vi "Change temperature with fixed current.vi"() -> ()   [LabVIEW 2013]
uses:
  <vilib>/Analysis/NI_AALBase.lvlib
panel:
  out "Variance":dbl[](array[numeric]) format="%#.2g"
  out "SD":dbl[](array[numeric]) format="%#.2g"
  out "Mean":dbl[](array[numeric]) format="%#.2f"
  out "variance":dbl format="%0.2f"
  out "standard deviation":dbl format="%0.2f"
  out "mean":dbl format="%0.2f"
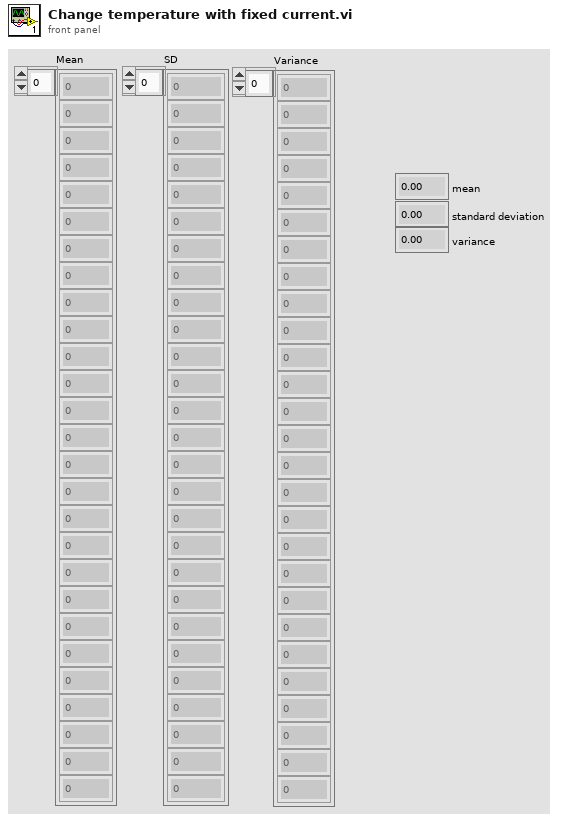
[diagram p1: front panel]
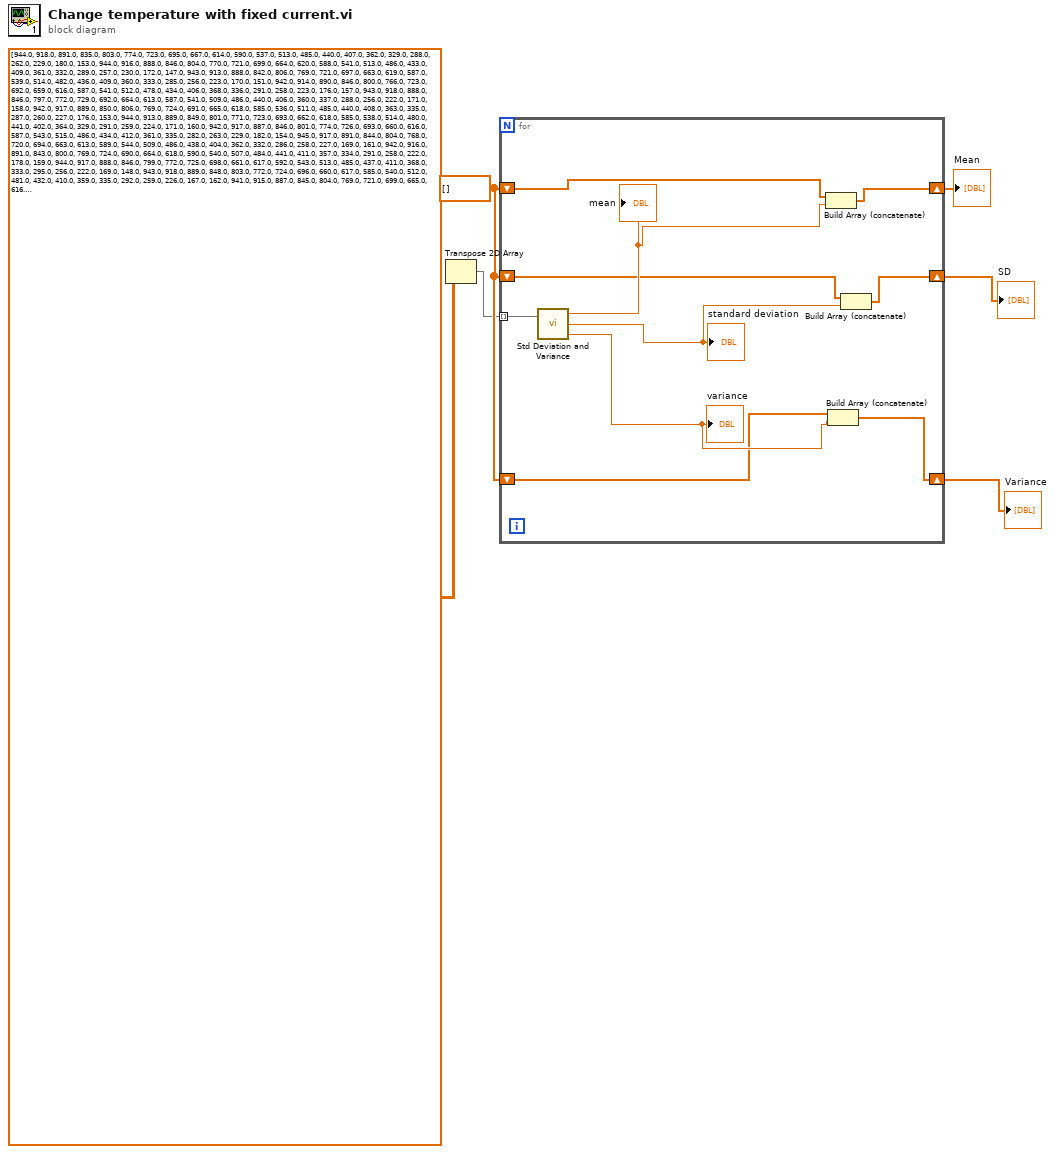
[diagram p0: block diagram]
diagram:
  w6 = dbl[] []
  n1 = Transpose 2D Array(2D array=dbl[][] [[944.0, 918.0, 891.0, 835.0, 803.0, 774.0, 723.0, 695.0, 667.0, 614.0, 590.0, 537.0, 513.0, 485.0, 440.0, 407.0, 362.0, 329.0, 288.0, 262.0, 229.0, 180.0, 153.0], [944.0, 916.0, 888.0, 846.0, 804.0, 770.0, 721.0, 699.0, 664.0, 620.0, 588.0, 541.0, 513.0, 486.0, 433.0, 409.0, 361.0, 332.0, 289.0, 257.0, 230.0, 172.0, 147.0], [943.0, 913.0, 888.0, 842.0, 806.0, 769.0, 721.0, 697.0, 663.0, 619.0, 587.0, 539.0, 514.0, 482.0, 436.0, 409.0, 360.0, 333.0, 285.0, 256.0, 223.0, 170.0, 151.0], [942.0, 914.0, 890.0, 846.0, 800.0, 766.0, 723.0, 692.0, 659.0, 616.0, 587.0, 541.0, 512.0, 478.0, 434.0, 406.0, 368.0, 336.0, 291.0, 258.0, 223.0, 176.0, 157.0], [943.0, 918.0, 888.0, 846.0, 797.0, 772.0, 729.0, 692.0, 664.0, 613.0, 587.0, 541.0, 509.0, 486.0, 440.0, 406.0, 360.0, 337.0, 288.0, 256.0, 222.0, 171.0, 158.0], [942.0, 917.0, 889.0, 850.0, 806.0, 769.0, 724.0, 691.0, 665.0, 618.0, 585.0, 536.0, 511.0, 485.0, 440.0, 408.0, 363.0, 335.0, 287.0, 260.0, 227.0, 176.0, 153.0], [944.0, 913.0, 889.0, 849.0, 801.0, 771.0, 723.0, 693.0, 662.0, 618.0, 585.0, 538.0, 514.0, 480.0, 441.0, 402.0, 364.0, 329.0, 291.0, 259.0, 224.0, 171.0, 160.0], [942.0, 917.0, 887.0, 846.0, 801.0, 774.0, 726.0, 693.0, 660.0, 616.0, 587.0, 543.0, 515.0, 486.0, 434.0, 412.0, 361.0, 335.0, 282.0, 263.0, 229.0, 182.0, 154.0], [945.0, 917.0, 891.0, 844.0, 804.0, 768.0, 720.0, 694.0, 663.0, 613.0, 589.0, 544.0, 509.0, 486.0, 438.0, 404.0, 362.0, 332.0, 286.0, 258.0, 227.0, 169.0, 161.0], [942.0, 916.0, 891.0, 843.0, 800.0, 769.0, 724.0, 690.0, 664.0, 618.0, 590.0, 540.0, 507.0, 484.0, 441.0, 411.0, 357.0, 334.0, 291.0, 258.0, 222.0, 178.0, 159.0], [944.0, 917.0, 888.0, 846.0, 799.0, 772.0, 725.0, 698.0, 661.0, 617.0, 592.0, 543.0, 513.0, 485.0, 437.0, 411.0, 368.0, 333.0, 295.0, 256.0, 222.0, 169.0, 148.0], [943.0, 918.0, 889.0, 848.0, 803.0, 772.0, 724.0, 696.0, 660.0, 617.0, 585.0, 540.0, 512.0, 481.0, 432.0, 410.0, 359.0, 335.0, 292.0, 259.0, 226.0, 167.0, 162.0], [941.0, 915.0, 887.0, 845.0, 804.0, 769.0, 721.0, 699.0, 665.0, 616.0, 588.0, 540.0, 512.0, 482.0, 437.0, 406.0, 367.0, 332.0, 286.0, 262.0, 217.0, 178.0, 159.0], [941.0, 916.0, 891.0, 848.0, 805.0, 771.0, 724.0, 693.0, 664.0, 613.0, 586.0, 535.0, 514.0, 483.0, 441.0, 407.0, 365.0, 335.0, 285.0, 262.0, 223.0, 180.0, 155.0], [942.0, 916.0, 887.0, 849.0, 800.0, 773.0, 722.0, 691.0, 667.0, 616.0, 589.0, 544.0, 509.0, 478.0, 442.0, 411.0, 359.0, 337.0, 287.0, 257.0, 227.0, 177.0, 157.0], [942.0, 918.0, 888.0, 845.0, 800.0, 769.0, 724.0, 695.0, 665.0, 622.0, 587.0, 541.0, 507.0, 481.0, 437.0, 408.0, 368.0, 336.0, 289.0, 258.0, 225.0, 174.0, 155.0], [941.0, 915.0, 887.0, 845.0, 806.0, 769.0, 726.0, 697.0, 663.0, 617.0, 588.0, 543.0, 512.0, 482.0, 443.0, 406.0, 360.0, 336.0, 285.0, 260.0, 228.0, 163.0, 155.0], [942.0, 918.0, 890.0, 845.0, 804.0, 768.0, 722.0, 691.0, 664.0, 617.0, 582.0, 543.0, 513.0, 484.0, 440.0, 407.0, 359.0, 335.0, 292.0, 260.0, 224.0, 179.0, 151.0], [940.0, 915.0, 890.0, 849.0, 803.0, 771.0, 725.0, 690.0, 663.0, 617.0, 588.0, 542.0, 509.0, 482.0, 434.0, 410.0, 365.0, 337.0, 289.0, 257.0, 226.0, 176.0, 155.0], [942.0, 919.0, 890.0, 846.0, 805.0, 771.0, 728.0, 690.0, 664.0, 613.0, 590.0, 543.0, 510.0, 475.0, 433.0, 410.0, 361.0, 336.0, 287.0, 253.0, 228.0, 173.0, 152.0], [944.0, 916.0, 889.0, 850.0, 804.0, 771.0, 724.0, 694.0, 662.0, 619.0, 589.0, 543.0, 505.0, 485.0, 441.0, 407.0, 369.0, 342.0, 285.0, 261.0, 224.0, 168.0, 157.0], [942.0, 915.0, 888.0, 847.0, 804.0, 770.0, 725.0, 693.0, 667.0, 615.0, 589.0, 539.0, 513.0, 483.0, 434.0, 405.0, 367.0, 328.0, 294.0, 262.0, 228.0, 176.0, 149.0], [941.0, 914.0, 887.0, 841.0, 803.0, 769.0, 723.0, 691.0, 665.0, 617.0, 585.0, 541.0, 516.0, 483.0, 441.0, 407.0, 360.0, 338.0, 289.0, 259.0, 219.0, 175.0, 150.0], [943.0, 916.0, 890.0, 849.0, 804.0, 769.0, 721.0, 696.0, 665.0, 619.0, 589.0, 540.0, 513.0, 484.0, 441.0, 411.0, 368.0, 331.0, 288.0, 249.0, 218.0, 183.0, 150.0], [945.0, 919.0, 888.0, 845.0, 799.0, 773.0, 720.0, 695.0, 662.0, 618.0, 588.0, 540.0, 515.0, 484.0, 440.0, 405.0, 365.0, 331.0, 293.0, 256.0, 218.0, 163.0, 155.0], [943.0, 917.0, 890.0, 844.0, 804.0, 770.0, 724.0, 692.0, 664.0, 618.0, 588.0, 533.0, 512.0, 484.0, 437.0, 414.0, 356.0, 331.0, 290.0, 253.0, 223.0, 163.0, 152.0], [943.0, 916.0, 889.0, 846.0, 804.0, 774.0, 723.0, 694.0, 664.0, 613.0, 587.0, 537.0, 506.0, 484.0, 432.0, 412.0, 367.0, 340.0, 282.0, 255.0, 229.0, 175.0, 154.0], [941.0, 916.0, 891.0, 848.0, 801.0, 770.0, 726.0, 696.0, 661.0, 617.0, 587.0, 541.0, 512.0, 477.0, 439.0, 406.0, 365.0, 339.0, 285.0, 259.0, 221.0, 164.0, 152.0], [941.0, 914.0, 890.0, 848.0, 804.0, 769.0, 724.0, 694.0, 660.0, 616.0, 587.0, 546.0, 514.0, 483.0, 434.0, 412.0, 362.0, 331.0, 286.0, 252.0, 231.0, 182.0, 156.0], [944.0, 916.0, 890.0, 846.0, 804.0, 772.0, 724.0, 693.0, 661.0, 619.0, 586.0, 544.0, 515.0, 483.0, 440.0, 408.0, 365.0, 336.0, 290.0, 254.0, 226.0, 172.0, 156.0], [943.0, 917.0, 890.0, 848.0, 805.0, 770.0, 722.0, 695.0, 663.0, 617.0, 585.0, 543.0, 513.0, 480.0, 436.0, 406.0, 365.0, 336.0, 290.0, 257.0, 226.0, 178.0, 150.0], [942.0, 917.0, 888.0, 845.0, 801.0, 774.0, 723.0, 696.0, 665.0, 615.0, 589.0, 541.0, 512.0, 484.0, 444.0, 410.0, 363.0, 338.0, 289.0, 257.0, 221.0, 179.0, 150.0], [942.0, 915.0, 890.0, 845.0, 803.0, 769.0, 726.0, 695.0, 664.0, 613.0, 587.0, 534.0, 511.0, 485.0, 442.0, 410.0, 369.0, 336.0, 278.0, 257.0, 224.0, 170.0, 158.0], [941.0, 916.0, 887.0, 851.0, 799.0, 770.0, 722.0, 694.0, 660.0, 609.0, 587.0, 541.0, 517.0, 484.0, 435.0, 412.0, 368.0, 340.0, 286.0, 255.0, 224.0, 179.0, 156.0], [942.0, 915.0, 888.0, 846.0, 801.0, 769.0, 724.0, 695.0, 662.0, 618.0, 588.0, 541.0, 508.0, 483.0, 434.0, 412.0, 368.0, 338.0, 288.0, 261.0, 218.0, 167.0, 156.0], [942.0, 915.0, 891.0, 850.0, 801.0, 769.0, 718.0, 690.0, 661.0, 617.0, 587.0, 542.0, 510.0, 482.0, 434.0, 413.0, 368.0, 339.0, 287.0, 255.0, 226.0, 170.0, 147.0], [940.0, 916.0, 891.0, 848.0, 804.0, 772.0, 724.0, 695.0, 664.0, 622.0, 579.0, 541.0, 509.0, 484.0, 443.0, 407.0, 365.0, 336.0, 289.0, 262.0, 224.0, 179.0, 151.0], [942.0, 916.0, 889.0, 850.0, 801.0, 768.0, 722.0, 691.0, 663.0, 617.0, 585.0, 543.0, 513.0, 482.0, 436.0, 409.0, 364.0, 333.0, 289.0, 255.0, 221.0, 176.0, 156.0], [943.0, 919.0, 889.0, 848.0, 801.0, 770.0, 721.0, 692.0, 662.0, 615.0, 585.0, 536.0, 510.0, 481.0, 442.0, 406.0, 362.0, 335.0, 290.0, 256.0, 228.0, 174.0, 156.0], [943.0, 916.0, 887.0, 850.0, 801.0, 772.0, 724.0, 693.0, 667.0, 614.0, 585.0, 544.0, 505.0, 481.0, 434.0, 412.0, 368.0, 339.0, 288.0, 263.0, 223.0, 179.0, 160.0], [941.0, 917.0, 890.0, 851.0, 802.0, 767.0, 726.0, 690.0, 662.0, 619.0, 583.0, 545.0, 514.0, 483.0, 442.0, 411.0, 360.0, 329.0, 289.0, 257.0, 223.0, 162.0, 152.0], [942.0, 916.0, 890.0, 844.0, 798.0, 770.0, 726.0, 692.0, 665.0, 612.0, 585.0, 542.0, 515.0, 481.0, 440.0, 412.0, 360.0, 339.0, 286.0, 258.0, 230.0, 171.0, 155.0], [943.0, 917.0, 888.0, 848.0, 801.0, 769.0, 728.0, 695.0, 661.0, 615.0, 584.0, 543.0, 504.0, 485.0, 439.0, 412.0, 369.0, 337.0, 286.0, 258.0, 224.0, 173.0, 155.0], [942.0, 915.0, 887.0, 845.0, 801.0, 776.0, 728.0, 696.0, 664.0, 616.0, 590.0, 540.0, 511.0, 482.0, 439.0, 412.0, 369.0, 337.0, 287.0, 258.0, 229.0, 167.0, 151.0], [942.0, 916.0, 890.0, 848.0, 804.0, 770.0, 724.0, 695.0, 659.0, 615.0, 587.0, 540.0, 510.0, 480.0, 441.0, 408.0, 359.0, 332.0, 290.0, 261.0, 229.0, 171.0, 155.0], [943.0, 918.0, 891.0, 850.0, 800.0, 770.0, 726.0, 695.0, 662.0, 614.0, 581.0, 547.0, 513.0, 484.0, 441.0, 408.0, 367.0, 336.0, 286.0, 257.0, 221.0, 174.0, 156.0], [945.0, 914.0, 887.0, 850.0, 802.0, 771.0, 726.0, 699.0, 663.0, 615.0, 590.0, 543.0, 513.0, 482.0, 434.0, 414.0, 359.0, 337.0, 284.0, 248.0, 219.0, 180.0, 149.0], [942.0, 915.0, 891.0, 849.0, 804.0, 771.0, 720.0, 690.0, 664.0, 616.0, 588.0, 546.0, 513.0, 477.0, 436.0, 414.0, 367.0, 331.0, 288.0, 255.0, 225.0, 169.0, 154.0], [943.0, 918.0, 890.0, 846.0, 801.0, 770.0, 725.0, 690.0, 662.0, 620.0, 592.0, 543.0, 509.0, 485.0, 438.0, 411.0, 368.0, 332.0, 286.0, 262.0, 223.0, 180.0, 159.0], [940.0, 915.0, 891.0, 849.0, 806.0, 774.0, 726.0, 694.0, 664.0, 618.0, 589.0, 544.0, 515.0, 483.0, 434.0, 412.0, 365.0, 334.0, 285.0, 251.0, 230.0, 172.0, 152.0], [941.0, 918.0, 891.0, 845.0, 798.0, 771.0, 721.0, 700.0, 667.0, 617.0, 588.0, 545.0, 514.0, 477.0, 442.0, 406.0, 365.0, 336.0, 290.0, 255.0, 231.0, 183.0, 148.0], [942.0, 918.0, 889.0, 845.0, 804.0, 773.0, 721.0, 696.0, 665.0, 616.0, 588.0, 545.0, 507.0, 480.0, 438.0, 415.0, 367.0, 335.0, 290.0, 261.0, 222.0, 178.0, 145.0]] ("array 2")) -> (transposed array=w1:dbl[][])
  n2 = for {
    tunnel: w1 -> [w16] mode=indexing
    shift-right: [w15] -> w5
    shift-left: w6 -> [w13]
    shift-right: [w11] -> w4
    shift-left: w6 -> [w10]
    shift-right: [w7] -> w3
    shift-left: w6 -> [w8]
    n3 = call <vilib>:"Std Deviation and Variance.vi"("X"=w16) -> ("mean"=w14:dbl, "standard deviation"=w12:dbl, "variance"=w9:dbl)  [unwired: 1 in]
    "mean" <- w14
    "standard deviation" <- w12
    "variance" <- w9
    n4 = Build Array (concatenate)(w13, w14) -> (w15:dbl[])
    n5 = Build Array (concatenate)(w8, w9) -> (w7:dbl[])
    n6 = Build Array (concatenate)(w10, w12) -> (w11:dbl[])
  }
  "Mean" <- w5
  "SD" <- w4
  "Variance" <- w3
